vi "Get.vi"(8 "error in (no error)":errorcluster, 11 "Thread Name":string) -> (0 "error out":errorcluster, 1 "Found?":bool, 2 "Generic VI Reference":refnum<vi>, 3 "VI Reference":variant)   [LabVIEW 2018, in "Thread.lvlib"]
uses:
  Thread.lvlib
  Cache Action.ctl
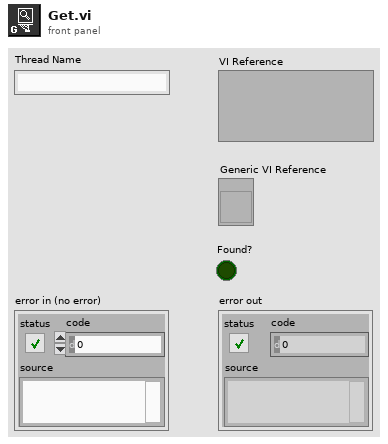
[diagram p1: front panel]
types:
  T1 = typedef "Thread.lvlib/Cache Action.ctl" = enum8{"noop", "get", "add", "remove", "remove_by_ref"}
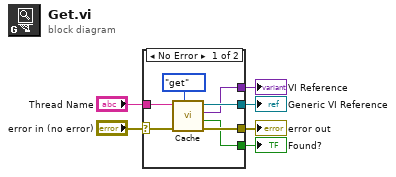
[diagram p0: block diagram]
diagram:
  n1 = case shown="No Error" "error in (no error)" {
    selector: "error in (no error)" -> [w12 w14]
    tunnel: [w10 w14] -> w5
    tunnel: [w8 _] -> w4
    tunnel: [w9 _] -> w3
    tunnel: "Thread Name" -> [w11 _]
    tunnel: [w7 _] -> w1
    frame No Error {
      n2 = call "Cache.vi"("Action"=Cache_Action."get", "error in (no error)"=w12, "Thread Name"=w11) -> ("error out"=w10:errorcluster, "Found?"=w7:bool, "VI out"=w8:variant, "Generic VI out"=w9:refnum<vi>)  [unwired: 4 in, 1 out]
    }
    frame Error {
    }
  }
  "error out" <- w5
  "Generic VI Reference" <- w3
  "VI Reference" <- w4
  "Found?" <- w1
